vi "Valve1DI1DO_CheckAlarms.vi"(11 "ValveState":T1) -> ()   [LabVIEW 2019]
uses:
  TypeDef/ValveState.ctl
  TypeDef/Alarms_1DO1DI.ctl
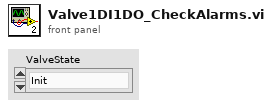
[diagram p1: front panel]
types:
  T1 = typedef "ValveState.ctl" = enum16{"Init", "Close", "Opening", "Open", "Closing"}
  T2 = typedef "Alarms_1DO1DI.ctl" = cluster{"Unsheduled open":bool, "Unsheduled close":bool, "Timeout open":bool, "Timeout close":bool}
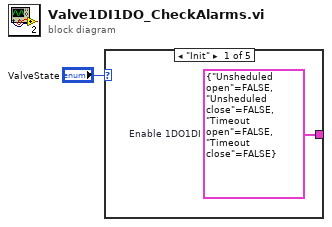
[diagram p0: block diagram]
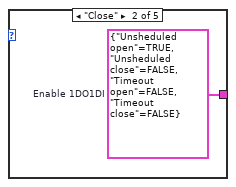
[diagram p2: hidden frame]
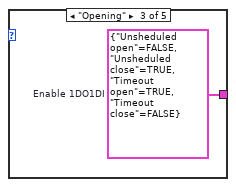
[diagram p3: hidden frame]
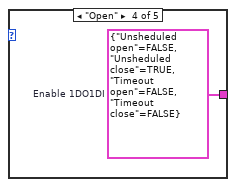
[diagram p4: hidden frame]
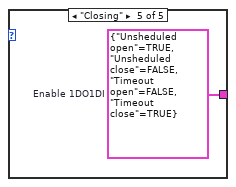
[diagram p5: hidden frame]
diagram:
  n1 = case shown="\"Init\"" "ValveState" {
    tunnel: [w2 w3 w4 w5 w6] -> _
    frame "Init" {
      w2 = T2 {"Unsheduled open"=FALSE, "Unsheduled close"=FALSE, "Timeout open"=FALSE, "Timeout close"=FALSE}  # Enable 1DO1DI
    }
    frame "Close" {
      w3 = T2 {"Unsheduled open"=TRUE, "Unsheduled close"=FALSE, "Timeout open"=FALSE, "Timeout close"=FALSE}  # Enable 1DO1DI
    }
    frame "Opening" {
      w4 = T2 {"Unsheduled open"=FALSE, "Unsheduled close"=TRUE, "Timeout open"=TRUE, "Timeout close"=FALSE}  # Enable 1DO1DI
    }
    frame "Open" {
      w5 = T2 {"Unsheduled open"=FALSE, "Unsheduled close"=TRUE, "Timeout open"=FALSE, "Timeout close"=FALSE}  # Enable 1DO1DI
    }
    frame "Closing" {
      w6 = T2 {"Unsheduled open"=TRUE, "Unsheduled close"=FALSE, "Timeout open"=FALSE, "Timeout close"=TRUE}  # Enable 1DO1DI
    }
  }
